vi "DHTxx Test Basic.vi"() -> ()   [LabVIEW 2014, in "ESP8266 WiFi Wrapper.lvlib"]
uses:
  <vilib>/Aledyne-TSXperts/Arduino Compatible Compiler for LabVIEW/addons/ESP8266 WiFi Wrapper/ESP8266 WiFi Wrapper.lvlib
panel:
  out "Temperature":dbl
  in  "Error In":errorcluster
  out "Error Out":errorcluster
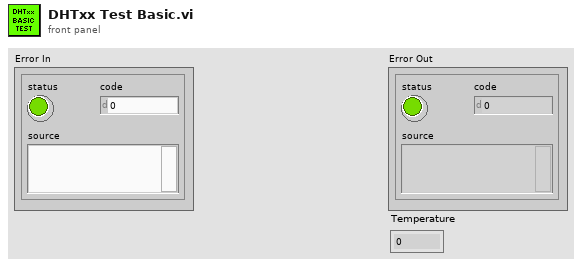
[diagram p1: front panel]
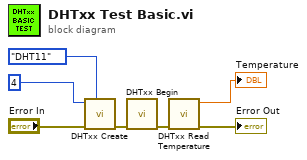
[diagram p0: block diagram]
diagram:
  n1 = call <vilib>:"DHTxx Create.vi"("DHT Type"=enum16{"DHT11", "DHT21", "DHT22"}."DHT11", "Error In"="Error In", "DHT pin"=u8 4) -> ("Error Out"=w5:errorcluster)  [unwired: 8 in]
  n2 = call <vilib>:"DHTxx Begin.vi"("Error In"=w5) -> ("Error Out"=w4:errorcluster)  [unwired: 10 in]
  n3 = call <vilib>:"DHTxx Read Temperature.vi"("Error In"=w4) -> ("Error Out"=→"Error Out":errorcluster, "Temperature"=→"Temperature":dbl)  [unwired: 9 in]
